vi "Send_control_char_and_STOP.vi"(8 "Select COM port":refnum<visa-resource-name>="COM3", 9 "STOP":bool, 10 "Char to send":string="b", 11 "Send Char":bool) -> ()   [LabVIEW 2012]
panel:
  in  "Select COM port":refnum<visa-resource-name>="COM3"
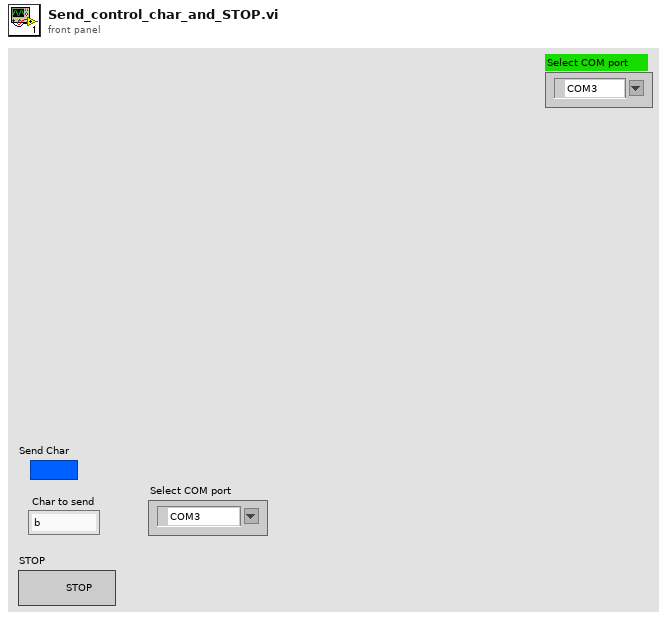
[diagram p1: front panel]
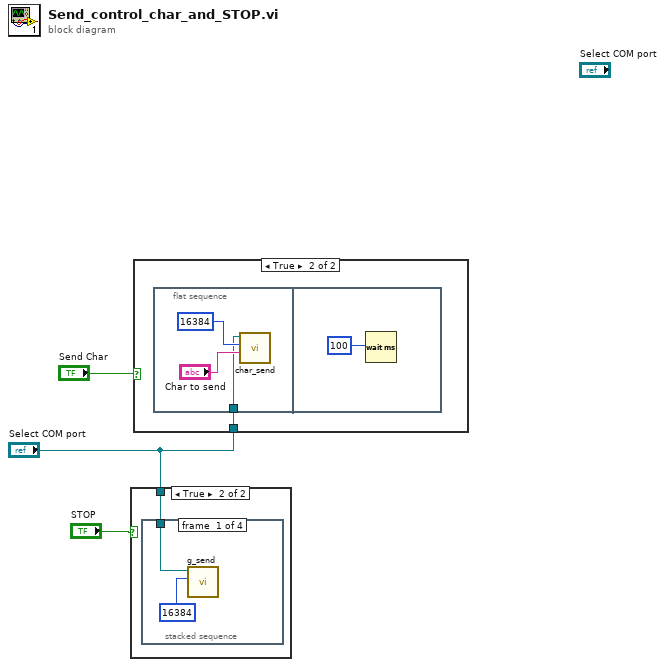
[diagram p0: block diagram]
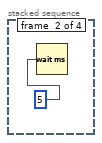
[diagram p4: hidden frame]
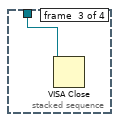
[diagram p5: hidden frame]
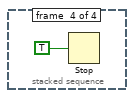
[diagram p6: hidden frame]
diagram:
  n1 = case shown="True" "STOP" {
    tunnel: "Select COM port" -> [_ w4]
    frame False {
    }
    frame True {
      n2 = stacked-sequence {
        tunnel: w4 -> [w6 _ w8 _]
        frame #0 {
          n3 = call "g_send.vi"("Input buffer size"=16384, "USB Interface Name"=w6) -> ()  [unwired: 9 in, 1 out]
        }
        frame #1 {
          n4 = Wait (ms)(milliseconds to wait=5) -> ()  [unwired: 1 out]
        }
        frame #2 {
          n5 = VISA Close(VISA resource name=w8) -> ()  [unwired: 1 in, 1 out]
        }
        frame #3 {
          n6 = Stop(stop? (T)=TRUE ("Stop? (T)")) -> ()
        }
      }
    }
  }
  n7 = case shown="True" "Send Char" {
    tunnel: "Select COM port" -> [_ w10]
    frame False {
    }
    frame True {
      n8 = flat-sequence {
        tunnel: w10 -> [w11]
        frame #0 {
          n9 = call "char_send.vi"("Char to send"="Char to send", "Input buffer size"=16384, "USB Interface Name"=w11) -> ()  [unwired: 9 in]
        }
        frame #1 {
          n10 = Wait (ms)(milliseconds to wait=100) -> ()  [unwired: 1 out]
        }
      }
    }
  }
